vi "Store Actors.vi"(8 "error in (no error)":errorcluster, 9 "Actor Paths":path[](array[path]), 10 "Actors":string[](array[string]), 11 "INI Store in":refnum<class "INI Store.lvclass">) -> (0 "error out":errorcluster, 3 "INI Store out":refnum<class "INI Store.lvclass">)   [LabVIEW 2020, in "Add Actor.lvlib" / "INI Store.lvclass"]
uses:
  INI Store.lvclass
  <resource>/dialog/lvconfig.llb/LV Config Write String.vi
  <resource>/dialog/lvconfig.llb/LV Config Write Pathlist.vi
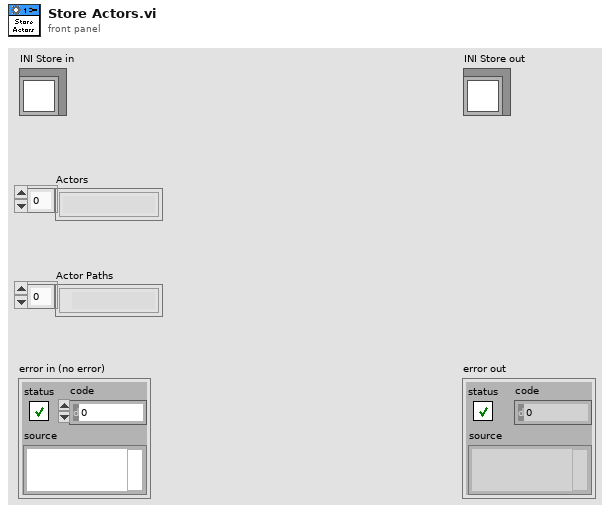
[diagram p1: front panel]
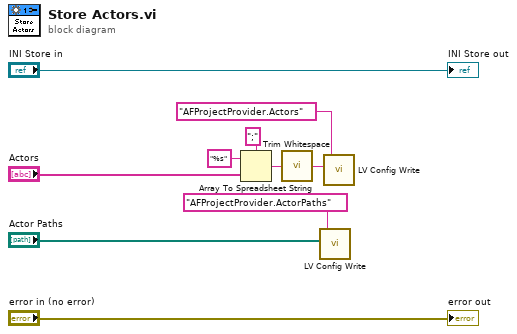
[diagram p0: block diagram]
diagram:
  n1 = Array To Spreadsheet String(delimiter (Tab)=";", array="Actors", 3:"%s" ("format string")) -> (spreadsheet string=w7:string)
  n2 = call <vilib>:"Trim Whitespace.vi"("string"=w7) -> ("trimmed string"=w10:string)  [unwired: 1 in]
  n3 = call-poly <resource>:"LV Config Write.vi"("value"="Actor Paths", "key"="AFProjectProvider.ActorPaths") -> ()  [unwired: 5 in, 1 out]
  n4 = call-poly <resource>:"LV Config Write.vi"("value"=w10, "key"="AFProjectProvider.Actors") -> ()  [unwired: 5 in, 1 out]
  "error out" <- "error in (no error)"
  "INI Store out" <- "INI Store in"
